vi "gen_sine_function.vi"(8 "error in (no error)":errorcluster, 10 "z signal graph ref":refnum<vi>, 11 "TrajectoryAK101022Resonance in":refnum<class "TrajectoryAK101022Resonance.lvclass">) -> (0 "error out":errorcluster, 1 "z-frequency":dbl[unit], 2 "z points":dbl[unit][](array[numeric]), 3 "TrajectoryAK101022Resonance out":refnum<class "TrajectoryAK101022Resonance.lvclass">)   [LabVIEW 2010, in "TrajectoryAK101022Resonance.lvclass"]
uses:
  TrajectoryAK101022Resonance.lvclass
  FPGAWrapper/FPGAWrapperAK101022Resonance/FPGAWrapperAK101022Resonance/FPGAWrapperAK101022Resonance.lvclass
  TrajectoryAK101022Resonance.lvclass/TrajectoryAK101022Resonance.ctl
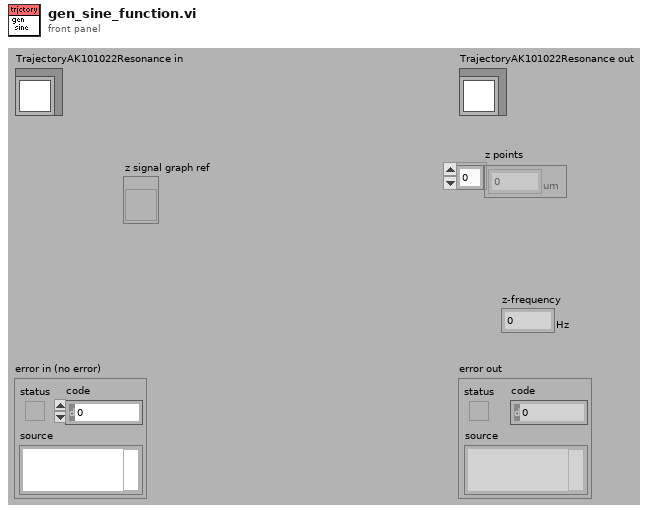
[diagram p1: front panel]
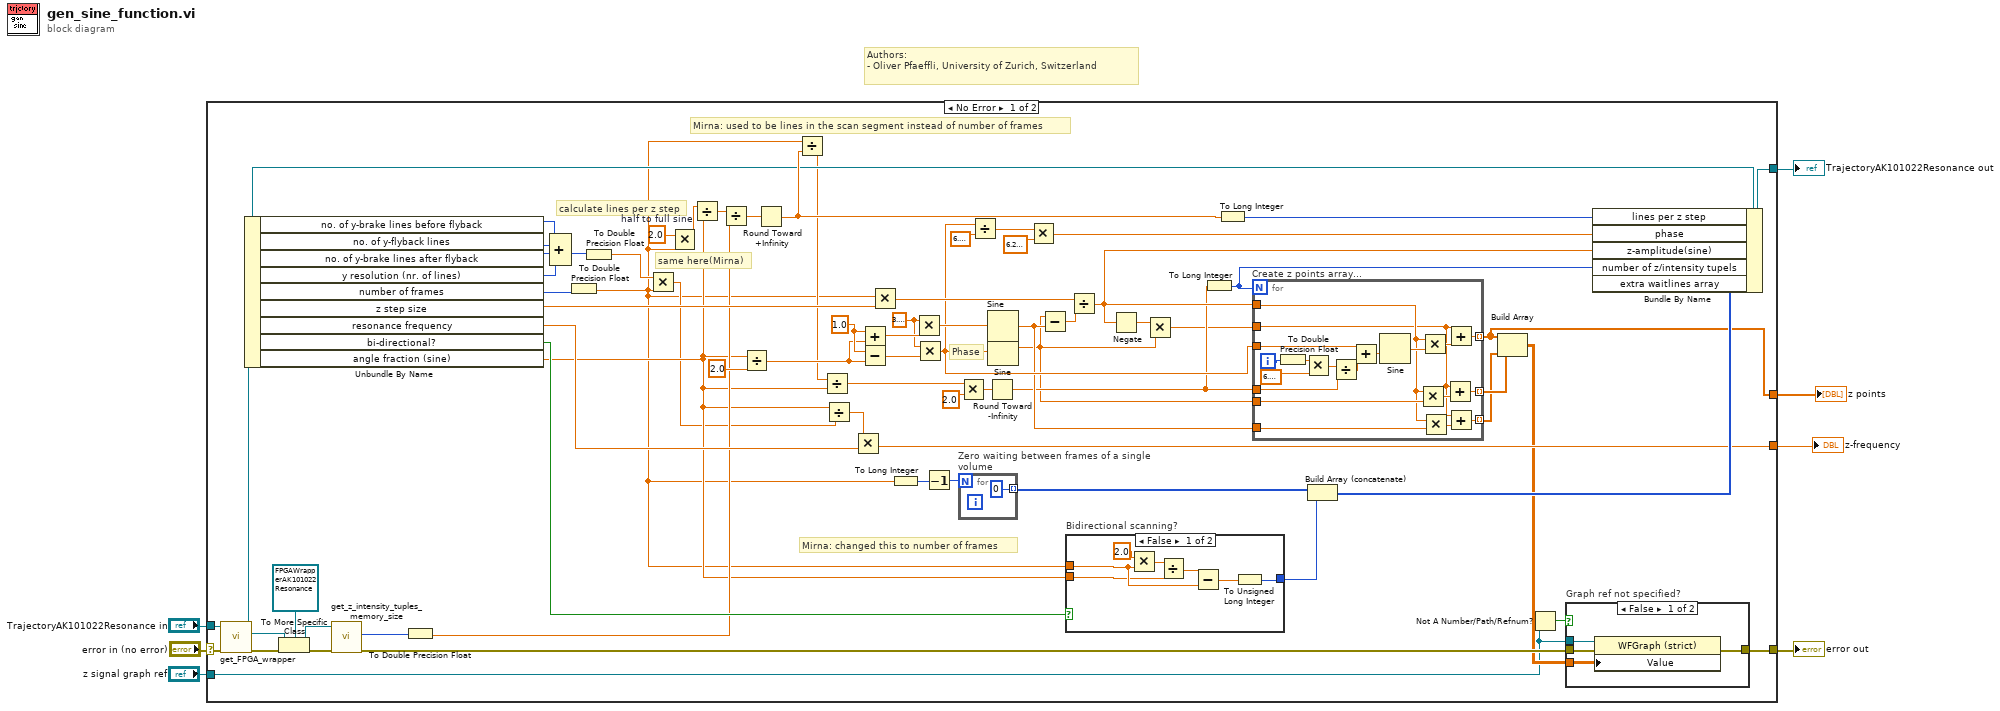
[diagram p0: block diagram]
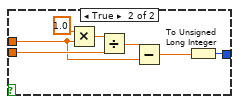
[diagram p3: hidden frame]
diagram:
  # "Authors: \n- Oliver Pfaeffli, University of Zurich, Switzerland"
  n1 = case shown="No Error" "error in (no error)" {
    selector: "error in (no error)" -> [w44 w118]
    tunnel: [w18 w118] -> w6
    tunnel: [w77 w117] -> w5
    tunnel: "TrajectoryAK101022Resonance in" -> [w43 w117]
    tunnel: [w21 _] -> w3
    tunnel: "z signal graph ref" -> [w16 _]
    tunnel: [w14 _] -> w1
    frame No Error {
      w55 = 2.0  # half to full sine
      w75 = 3.141592653589793
      w62 = 1.0
      # "Mirna: changed this to number of frames"
      # "same here(Mirna)"
      # "Mirna: used to be lines in the scan segment instead of number of frames"
      # "calculate lines per z step"
      # "Phase"
      n2 = call-dynamic "get_FPGA_wrapper.vi"("error in (no error)"=w44, "TrajectoryMG100122GenericFPGA in"=w43) -> ("error out"=w40:errorcluster, "GenericFPGAWrapper.lvclass"=w41:refnum<class "GenericFPGAWrapper.lvclass">, "TrajectoryMG100122GenericFPGA out"=w42:refnum<class "TrajectoryAK101022Resonance.lvclass">)  [unwired: 7 in]
      n3 = Unbundle By Name(w42) -> ("no. of y-brake lines before flyback"=w51:i32, "no. of y-flyback lines"=w50:i32, "no. of y-brake lines after flyback"=w49:i32, "y resolution (nr. of lines)"=w28:i32, "number of frames"=w26:i32, "z step size"=w25:dbl[unit], "resonance frequency"=w29:dbl[unit], "bi-directional?"=w34:bool, "angle fraction (sine)"=w20:dbl)
      n4 = To More Specific Class(target class=refnum<class "FPGAWrapperAK101022Resonance.lvclass"> refnum ("FPGAWrapperAK101022Resonance.lvclass"), reference=w41, error in=w40) -> (specific class reference=w37:refnum<class "FPGAWrapperAK101022Resonance.lvclass">, error out=w39:errorcluster)
      n5 = call "get_z_intensity_tuples_memory_size.vi"("error in (no error)"=w39, "FPGAWrapperAK101022Resonance in"=w37) -> ("error out"=w19:errorcluster, "z/intensity memory size"=w36:i32)  [unwired: 7 in, 1 out]
      n6 = To Double Precision Float(number=w36) -> (double precision float=w24:dbl)
      n7 = Compound Arithmetic op=ADD(w51, w50, w49, w28) -> (w27:i32)
      n8 = To Double Precision Float(number=w26) -> (double precision float=w8:dbl)
      n9 = To Double Precision Float(number=w27) -> (double precision float=w59:dbl)
      n10 = Multiply(x=w59, y=w8) -> (x*y=w10:dbl)
      n11 = Multiply(x=w55, y=w8) -> (x*y=w54:dbl)
      n12 = Divide(x=w54, y=w20) -> (x/y=w56:dbl)
      n13 = Divide(x=w56, y=w24) -> (x/y=w58:dbl)
      n14 = Divide(x=w20, y=2.0) -> (x/y=w61:dbl)
      n15 = Round Toward +Infinity(x=w58) -> (ceil(x): smallest int >= x=w53:dbl)
      n16 = Divide(x=w8, y=w53) -> (x/y=w9:dbl)
      n17 = Divide(x=w9, y=w20) -> (x/y=w11:dbl)
      n18 = Divide(x=w20, y=w10) -> (x/y=w45:dbl)
      n19 = Multiply(x=w45, y=w29) -> (x*y=w21:dbl[unit])
      n20 = Add(x=w62, y=w61) -> (x+y=w76:dbl)
      n21 = Subtract(x=w62, y=w61) -> (x-y=w74:dbl)
      n22 = Multiply(x=w8, y=w25) -> (x*y=w71:dbl[unit])
      n23 = To Long Integer(number=w8) -> (32bit integer=w33:i32)
      n24 = Multiply(x=w75, y=w76) -> (x*y=w73:dbl)
      n25 = Multiply(x=w75, y=w74) -> (x*y=w66:dbl)
      n26 = Decrement(x=w33) -> (x-1=w32:i32)
      n27 = Multiply(x=w11, y=2.0) -> (x*y=w68:dbl)
      n28 = for "Zero waiting between frames of a single volume" {
        N: w32 -> [_]
        tunnel: [u32 0] -> w35 mode=indexing
      }
      n29 = Divide(x=w66, y=6.283185307179586) -> (x/y=w64:dbl)
      n30 = Round Toward -Infinity(1:w68) -> (0:w31:dbl)
      n31 = Sine(x=w73) -> (sin(x)=w48:dbl)
      n32 = Sine(x=w66) -> (sin(x)=w12:dbl)
      n33 = Multiply(x=w64, y=dbl[unit] 6.283185307179586) -> (x*y=w63:dbl[unit])
      n34 = Subtract(x=w12, y=w48) -> (x-y=w72:dbl)
      n35 = case "Bidirectional scanning?" shown="False" w34 {
        tunnel: w8 -> [w85 w91]
        tunnel: [w83 w96] -> w30
        tunnel: w20 -> [w84 w93]
        frame False {
          n36 = Multiply(x=2.0, y=w85) -> (x*y=w88:dbl)
          n37 = Divide(x=w88, y=w84) -> (x/y=w87:dbl)
          n38 = Subtract(x=w87, y=w85) -> (x-y=w86:dbl)
          n39 = To Unsigned Long Integer(number=w86) -> (unsigned 32bit integer=w83:u32)
        }
        frame True {
          n40 = Multiply(x=1.0, y=w91) -> (x*y=w94:dbl)
          n41 = Divide(x=w94, y=w93) -> (x/y=w92:dbl)
          n42 = Subtract(x=w92, y=w91) -> (x-y=w90:dbl)
          n43 = To Unsigned Long Integer(number=w90) -> (unsigned 32bit integer=w96:u32)
        }
      }
      n44 = Divide(x=w71, y=w72) -> (x/y=w52:dbl[unit])
      n45 = Negate(x=w52) -> (-x=w70:dbl[unit])
      n46 = Multiply(x=w70, y=w12) -> (x*y=w23:dbl[unit])
      n47 = To Long Integer(number=w31) -> (32bit integer=w13:i32)
      n48 = To Long Integer(number=w53) -> (32bit integer=w57:i32)
      n49 = for "Create z points array..." {
        N: w13 -> [_]
        tunnel: w31 -> [w115]
        tunnel: w52 -> [w102]
        tunnel: w66 -> [w108]
        tunnel: w23 -> [w101]
        tunnel: [w109] -> w14 mode=indexing
        tunnel: w12 -> [w105]
        tunnel: w48 -> [w99]
        tunnel: [w103] -> w47 mode=indexing
        tunnel: [w98] -> w46 mode=indexing
        i -> [w107]
        n50 = To Double Precision Float(number=w107) -> (double precision float=w106:dbl)
        n51 = Multiply(x=w106, y=6.283185307179586) -> (x*y=w116:dbl)
        n52 = Divide(x=w116, y=w115) -> (x/y=w111:dbl)
        n53 = Add(x=w108, y=w111) -> (x+y=w113:dbl)
        n54 = Sine(x=w113) -> (sin(x)=w112:dbl)
        n55 = Multiply(x=w102, y=w105) -> (x*y=w104:dbl[unit])
        n56 = Multiply(x=w102, y=w112) -> (x*y=w110:dbl[unit])
        n57 = Multiply(x=w102, y=w99) -> (x*y=w100:dbl[unit])
        n58 = Add(x=w101, y=w104) -> (x+y=w103:dbl[unit])
        n59 = Add(x=w101, y=w110) -> (x+y=w109:dbl[unit])
        n60 = Add(x=w101, y=w100) -> (x+y=w98:dbl[unit])
      }
      n61 = Build Array (concatenate)(w35, w30) -> (w22:u32[])
      n62 = Build Array(w14, w47, w46) -> (w17:dbl[unit][][])
      n63 = Not A Number/Path/Refnum?(number/path/refnum=w16) -> (NaN/Path/Refnum?=w15:bool)
      n64 = case "Graph ref not specified?" shown="False" w15 {
        tunnel: w19 -> [w81 w82]
        tunnel: [w80 w82] -> w18
        tunnel: w16 -> [w79 _]
        tunnel: w17 -> [w78 _]
        frame False {
          n65 = property class="WFGraph (strict)"(reference=w79, error in=w81, "Value"=w78) -> (error out=w80:errorcluster)  [unwired: 1 out]
        }
        frame True {
        }
      }
      n66 = Bundle By Name(cluster=w42, "lines per z step"=w57, "phase"=w63, "z-amplitude(sine)"=w52, "number of z/intensity tupels"=w13, "extra waitlines array"=w22) -> (w77:refnum<class "TrajectoryAK101022Resonance.lvclass">)
    }
    frame Error {
    }
  }
  "error out" <- w6
  "TrajectoryAK101022Resonance out" <- w5
  "z-frequency" <- w3
  "z points" <- w1
